vi "Main.vi"() -> ()   [LabVIEW 2017]
uses:
  Controls/Main_St.ctl
  Controls/Main_Loop_Data_Flow.ctl
  <vilib>/Utility/error.llb/DialogType.ctl
  <vilib>/Utility/config.llb/NI_LVConfig.lvlib
panel:
  in  "Recipe":bool
  in  "USER CREATER":bool
  in  "HARDWARE SETTING":bool
  in  "APPLICATION LAUNCH":bool
  in  "Login":bool
  out "Number of Monitor Connected":i32
  out "error out":errorcluster
  in  "Close":bool
  out "Machine Name":string
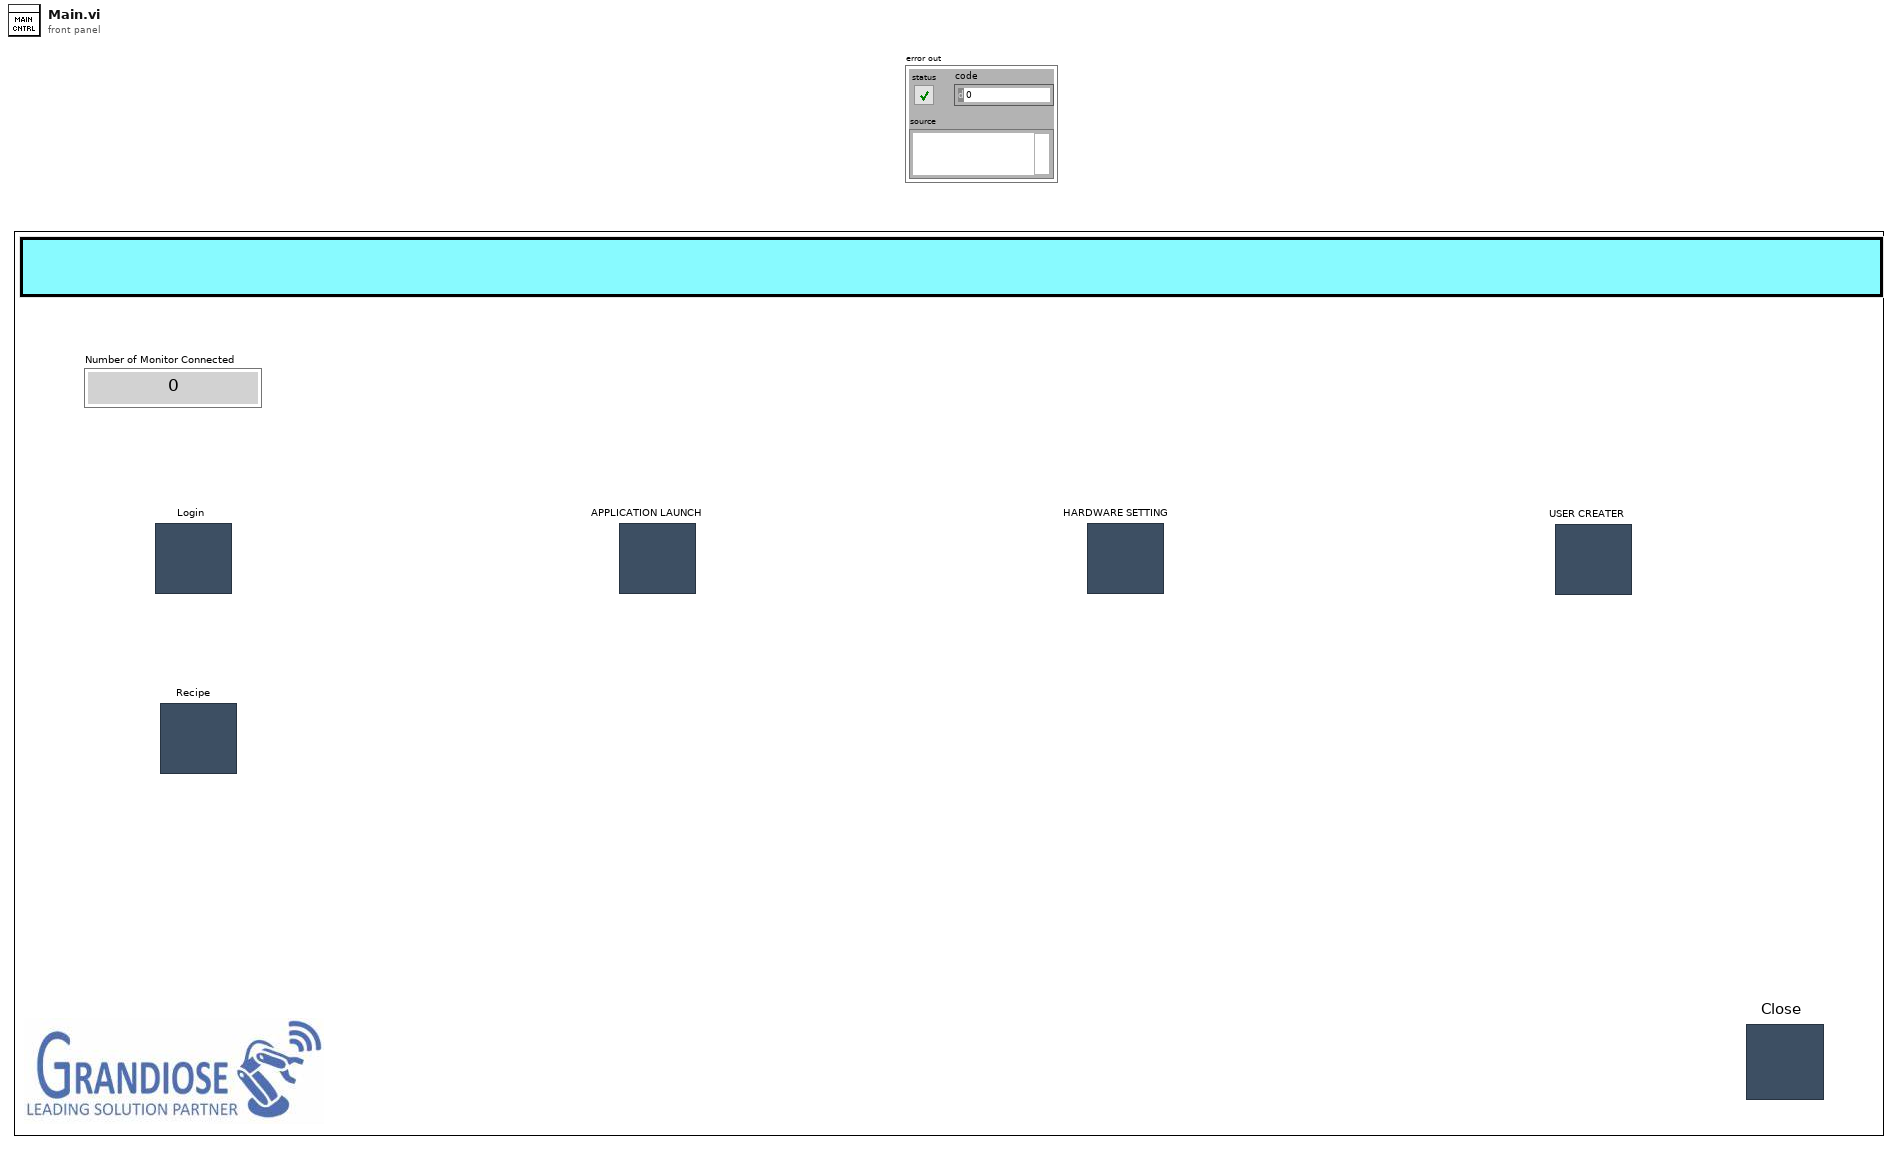
[diagram p1: front panel]
types:
  T1 = typedef "Main_Loop_Data_Flow.ctl" = cluster{"Hardware Setting":path, "Hardware":cluster{"Monitor Primary 1":u16, "Monitor 2":u16, "Monitor 3":u16, "Scanner IP":string, "Scanner 2":refnum<visa-resource-name>, "Scanner 3":refnum<visa-resource-name>, "Printer IP":string, "Printer 2":refnum<visa-resource-name>, "Printer 3":refnum<visa-resource-name>}, "SOP Path":path, "PNR Path":path, "PRN Data":string}
  T2 = typedef "Main_St.ctl" = enum16{"Int", "Int2", "Int3", "Wait", "Exit"}
  T3 = enum32{"Invalid", "Standard", "Closed", "Hidden", "Minimized", "Maximized"}
  T4 = typedef "DialogType.ctl" = u16
  T5 = enum8{"Enabled", "Disabled", "Disabled and Grayed Out"}
  T6 = enum32{"invalid app kind", "Development System", "Run Time System", "Student Edition", "Embedded LabVIEW", "Evaluation", "Custom"}
  T7 = cluster{"Monitor Primary 1":u16, "Monitor 2":u16, "Monitor 3":u16, "Scanner IP":string, "Scanner 2":refnum<visa-resource-name>, "Scanner 3":refnum<visa-resource-name>, "Printer IP":string, "Printer 2":refnum<visa-resource-name>, "Printer 3":refnum<visa-resource-name>}
  T8 = typedef "LVAllMonitorsDisplayTypeDef.ctl" = cluster{"Bounds":cluster{"Left":i16, "Top":i16, "Right":i16, "Bottom":i16}, "Depth":i16}[]
  T9 = typedef "NI_LVConfig.lvlib/Config Data RefNum.ctl" = refnum<k1>
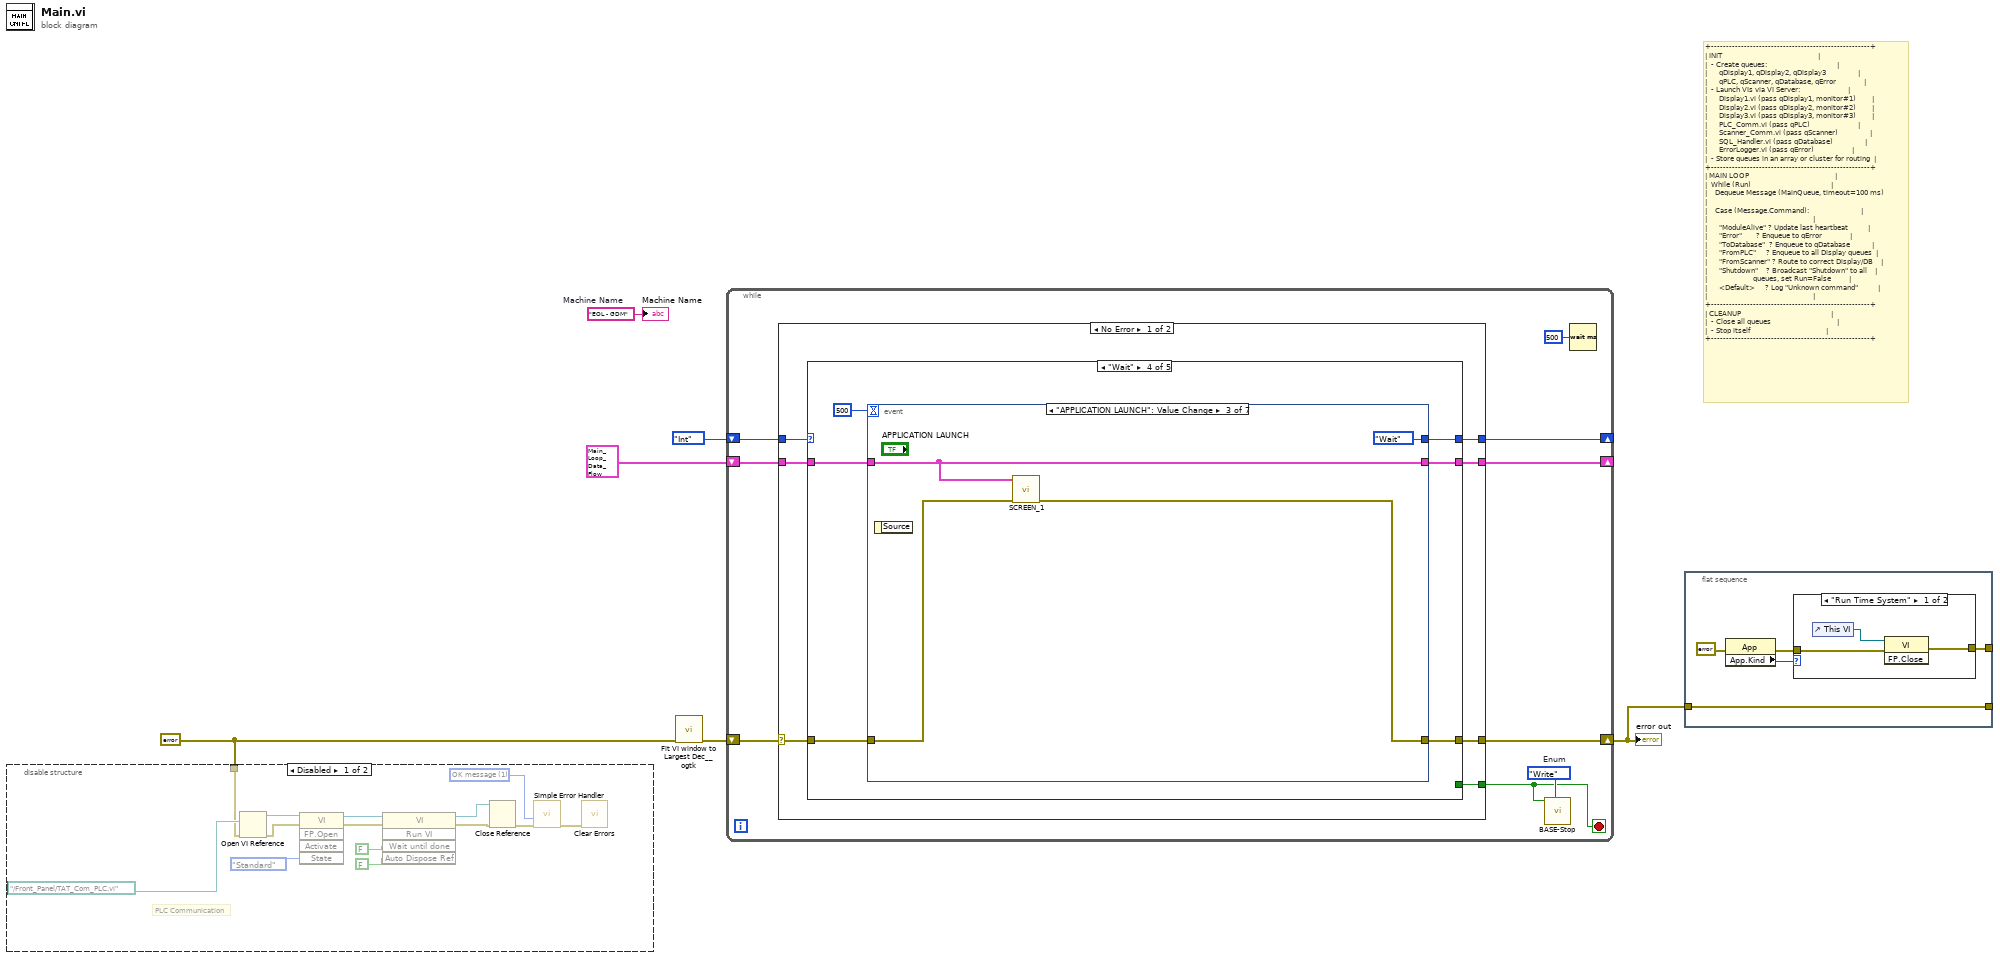
[diagram p0: block diagram]
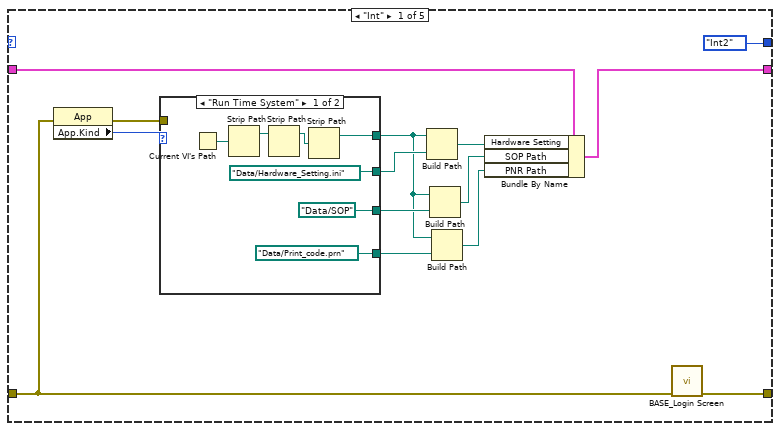
[diagram p4: hidden frame]
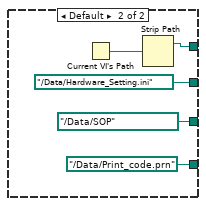
[diagram p5: hidden frame]
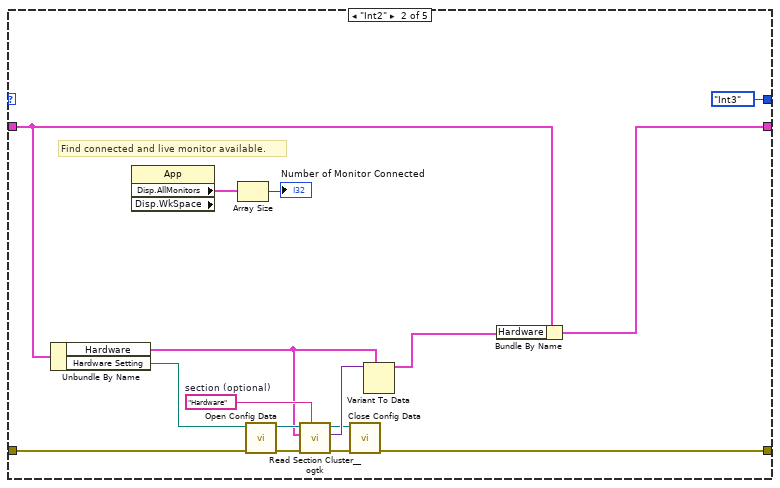
[diagram p6: hidden frame]
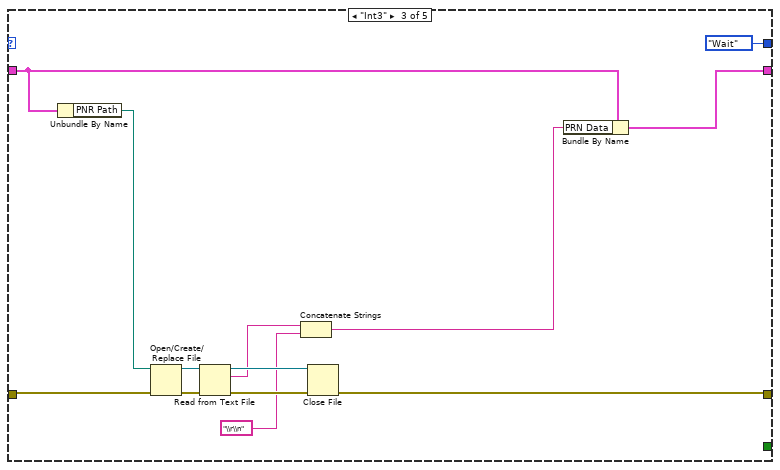
[diagram p7: hidden frame]
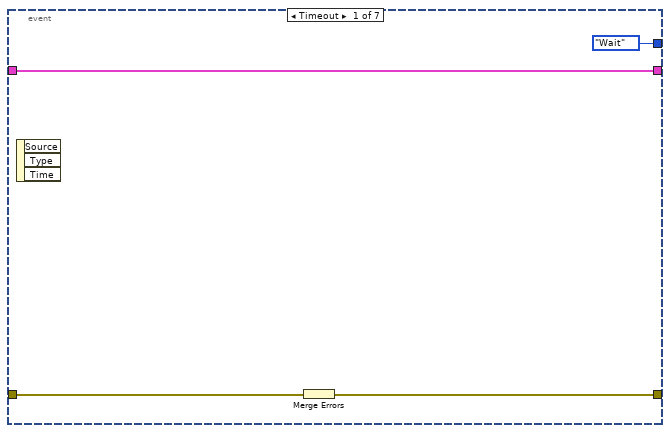
[diagram p8: hidden frame]
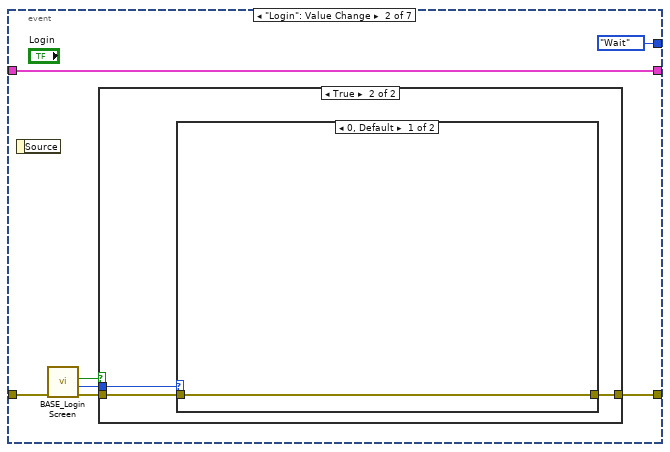
[diagram p9: hidden frame]
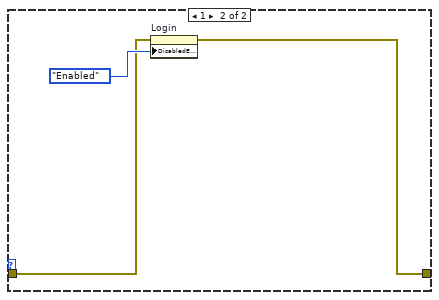
[diagram p11: hidden frame]
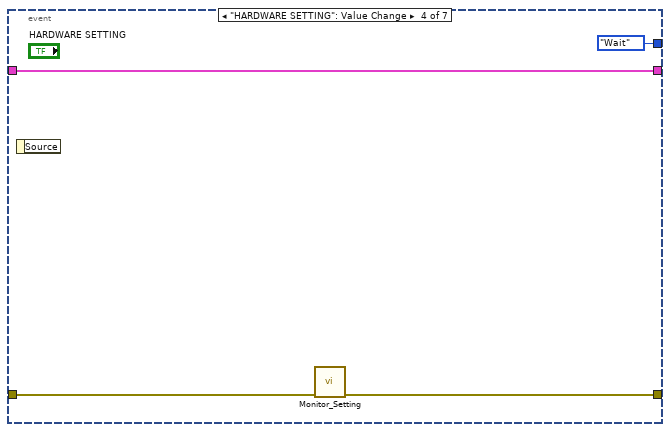
[diagram p12: hidden frame]
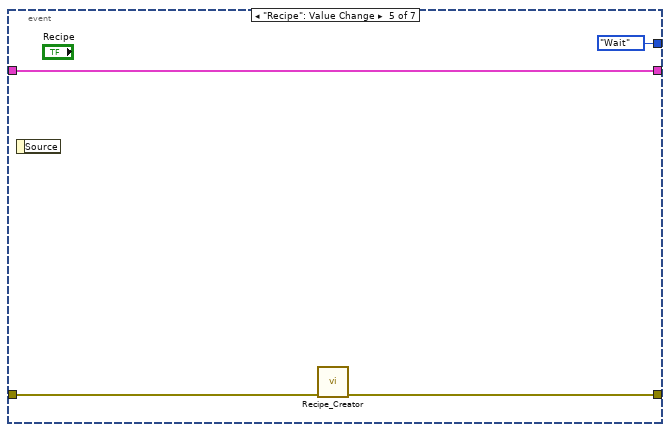
[diagram p13: hidden frame]
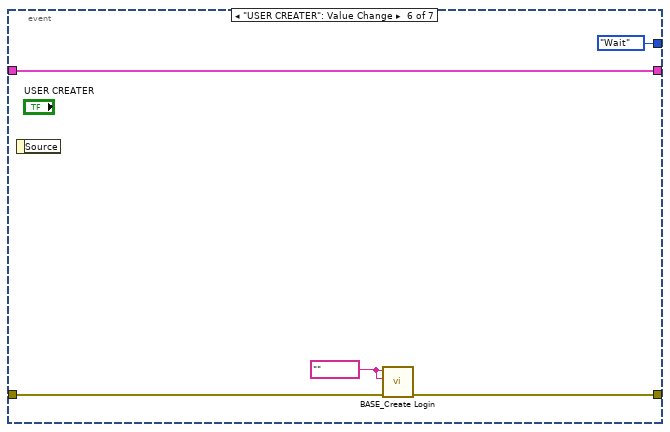
[diagram p14: hidden frame]
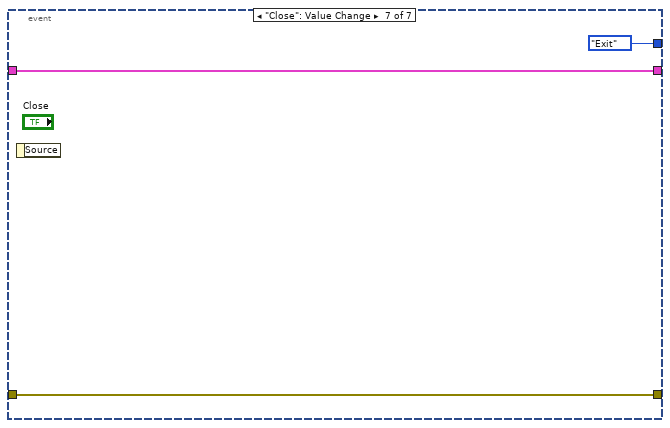
[diagram p15: hidden frame]
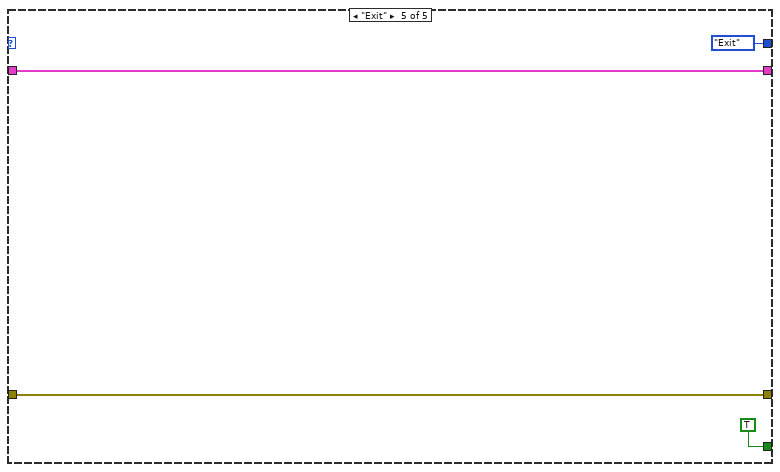
[diagram p16: hidden frame]
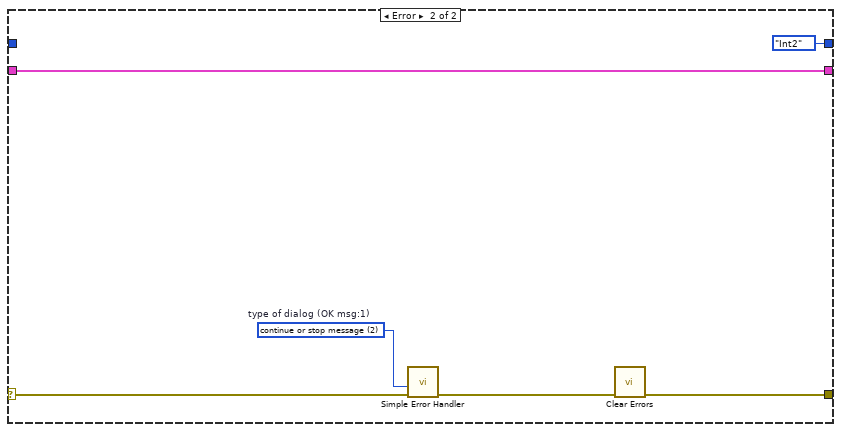
[diagram p17: hidden frame]
diagram:
  w3 = errorcluster {"status"=FALSE, "code"=0, "source"=""} ("error in (no error)")
  w6 = "EOL - GDM"  # Machine Name
  # "+-----------------------------------------------------+\n| INIT                                                |\n|  - Create queues:                                   |\n|      qDisplay1, qDisplay2, qDisplay3                |\n|      qPLC, qScanner, qDatabase, qError              |\n|  - Launch VIs via VI Server:                        |\n|      Display1.vi (pass qDisplay1, monitor#1)        |\n|      Display2.vi (pass qDisplay2, monitor#2)        |\n|      Display3.vi (pass qDisplay3, monitor#3)        |\n|      PLC_Comm.vi (pass qPLC)                        |\n|      Scanner_Comm.vi (pass qScanner)                |\n|      SQL_Handler.vi (pass qDatabase)                |\n|      ErrorLogger.vi (pass qError)                   |\n|  - Store queues in an array or cluster for routing  |\n+-----------------------------------------------------+\n| MAIN LOOP                                           |\n|  While (Run)                                        |\n|    Dequeue Message (MainQueue, timeout=100 ms)      |\n|    Case (Message.Command):                          |\n|                                                     |\n|      \"ModuleAlive\" ? Update last heartbeat          |\n|      \"Error\"       ? Enqueue to qError              |\n|      \"ToDatabase\"  ? Enqueue to qDatabase           |\n|      \"FromPLC\"     ? Enqueue to all Display queues  |\n|      \"FromScanner\" ? Route to correct Display/DB    |\n|      \"Shutdown\"    ? Broadcast \"Shutdown\" to all    |\n|                       queues, set Run=False         |\n|      <Default>     ? Log \"Unknown command\"          |\n|                                                     |\n+-----------------------------------------------------+\n| CLEANUP                                             |\n|  - Close all queues                                 |\n|  - Stop itself                                      |\n+-----------------------------------------------------+"
  n1 = disable-structure shown="Disabled" {
    disable-tunnel: w3 -> [w8 _]
    frame Disabled {
      w10 = T4 1 items=["no dialog", "OK message", "continue or stop message", "OK message + warnings", "continue/stop + warnings"] ("type of dialog (OK msg:1)")
      # "PLC Communication"
      n2 = Open VI Reference(vi path=path "../Front_Panel/TAT_Com_PLC.vi", error in (no error)=w8) -> (vi reference=w17:refnum<vi>, error out=w18:errorcluster)  [unwired: 4 in]
      n3 = invoke class="VI" method="FP.Open"(reference=w17, error in=w18, "State"=T3."Standard") -> (reference out=w20:refnum<vi>, error out=w19:errorcluster)  [unwired: 2 in, 3 out]
      n4 = invoke class="VI" method="Run VI"(reference=w20, error in=w19, "Wait until done"=FALSE ("Wait Until Done"), "Auto Dispose Ref"=FALSE ("Auto Dispose Reference")) -> (reference out=w7:refnum<vi>, error out=w16:errorcluster)  [unwired: 1 in, 3 out]
      n5 = Close Reference(reference=w7, error in (no error)=w16) -> (error out=w11:errorcluster)
      n6 = call <vilib>:"Simple Error Handler.vi"("type of dialog (OK msg:1)"=w10, "error in (no error)"=w11) -> ("error out"=w9:errorcluster)  [unwired: 3 in, 4 out]
      n7 = call <vilib>:"Clear Errors.vi"("error in (no error)"=w9) -> ()  [unwired: 5 in, 2 out]
    }
    frame Enabled {
    }
  }
  n8 = call <userlib>:"Fit VI window to Largest Dec__ogtk.vi"("error in (no error)"=w3) -> ("error out"=w5:errorcluster)  [unwired: 5 in, 1 out]
  n9 = while {
    shift-right: [w27] -> w1
    shift-left: w5 -> [w28]
    shift-right: [w23] -> _
    shift-left: Main_St."Int" -> [w26]
    shift-right: [w24] -> _
    shift-left: T1 {"Hardware Setting"=path "", "Hardware"={"Monitor Primary 1"=1, "Monitor 2"=2, "Monitor 3"=3, "Scanner IP"="", "Scanner 2"="", "Scanner 3"="", "Printer IP"="", "Printer 2"="", "Printer 3"=""}, "SOP Path"=path "", "PNR Path"=path "", "PRN Data"=""} -> [w25]
    stop <- w21 stop-if-true
    w22 = enum16{"Read", "Write"}."Write"  # Enum
    n10 = case shown="No Error" w28 {
      selector: w28 -> [w36 w146]
      tunnel: [w35 w141] -> w27
      tunnel: w26 -> [w34 _]
      tunnel: w25 -> [w33 w143]
      tunnel: [w32 w143] -> w24
      tunnel: [w31 Main_St."Int2"] -> w23
      tunnel: [w30 _] -> w21
      frame No Error {
        n11 = case shown="\"Wait\"" w34 {
          tunnel: w36 -> [w44 w71 w84 w97 w137]
          tunnel: [w43 w69 w83 w96 w137] -> w35
          tunnel: w33 -> [w47 w67 w81 w93 w139]
          tunnel: [w46 w66 w80 w92 w139] -> w32
          tunnel: [Main_St."Int2" Main_St."Int3" Main_St."Wait" w95 Main_St."Exit"] -> w31
          tunnel: [_ _ _ _ TRUE] -> w30
          frame "Int" {
            n12 = property class="App"(error in=w44) -> (error out=w50:errorcluster, "App.Kind"=w48:T6)  [unwired: 1 in, 1 out]
            n13 = case shown="\"Run Time System\"" w48 {
              tunnel: [path "Data/Hardware_Setting.ini" ("path") path "../Data/Hardware_Setting.ini" ("path")] -> w49
              tunnel: [w53 w60] -> w38
              tunnel: w50 -> [_ _]
              tunnel: [path "Data/SOP" ("path") path "../Data/SOP" ("path")] -> w41
              tunnel: [path "Data/Print_code.prn" ("path") path "../Data/Print_code.prn" ("path")] -> w39
              frame "Run Time System" {
                n14 = Current VI's Path() -> (path=w56:path)
                n15 = Strip Path(path=w56) -> (stripped path=w55:path)  [unwired: 1 out]
                n16 = Strip Path(path=w55) -> (stripped path=w54:path)  [unwired: 1 out]
                n17 = Strip Path(path=w54) -> (stripped path=w53:path)  [unwired: 1 out]
              }
              frame Default {
                n18 = Current VI's Path() -> (path=w61:path)
                n19 = Strip Path(path=w61) -> (stripped path=w60:path)  [unwired: 1 out]
              }
            }
            n20 = Build Path(base path=w38, name or relative path=w49) -> (appended path=w42:path)
            n21 = Build Path(base path=w38, name or relative path=w41) -> (appended path=w40:path)
            n22 = Build Path(base path=w38, name or relative path=w39) -> (appended path=w37:path)
            n23 = Bundle By Name(cluster=w47, "Hardware Setting"=w42, "SOP Path"=w40, "PNR Path"=w37) -> (w46:T1)
            n24 = call "BASE_Login Screen.vi"("Error In"=w44) -> ("error out"=w43:errorcluster)  [unwired: 7 in, 3 out]
          }
          frame "Int2" {
            w72 = "Hardware"  # section (optional)
            # "Find connected and live monitor available."
            n25 = Unbundle By Name(w67) -> ("Hardware"=w65:T7, "Hardware Setting"=w70:path)
            n26 = property class="App" props=["Disp.AllMonitors", "Disp.WkSpace"]() -> ("Disp.AllMonitors"=w64:T8)  [unwired: 2 in, 3 out]
            n27 = Array Size(array=w64) -> (size(s)=→"Number of Monitor Connected":i32)
            n28 = call <vilib>:"Open Config Data.vi"("error in (no error)"=w71, "configuration file path"=w70) -> ("error out"=w73:errorcluster, "refnum"=w76:T9)  [unwired: 7 in, 1 out]
            n29 = call <userlib>:"Read Section Cluster__ogtk.vi"("section (optional)"=w72, "error in (no error)"=w73, "Section Formatted Cluster Type"=w65, "refnum"=w76) -> ("error out"=w74:errorcluster, "Section Formatted Cluster"=w77:variant, "dup refnum"=w75:T9)  [unwired: 3 in, 2 out]
            n30 = call <vilib>:"Close Config Data.vi"("error in (no error)"=w74, "refnum"=w75) -> ("error out"=w69:errorcluster)  [unwired: 8 in, 1 out]
            n31 = Variant To Data(type=w65, Variant=w77) -> (data=w68:T7)  [unwired: 1 in, 1 out]
            n32 = Bundle By Name(cluster=w67, "Hardware"=w68) -> (w66:T1)
          }
          frame "Int3" {
            n33 = Unbundle By Name(w81) -> ("PNR Path"=w82:path)
            n34 = Open/Create/Replace File(file path (use dialog)=w82, error in=w84) -> (refnum out=w89:refnum<file>, error out=w88:errorcluster)  [unwired: 4 in, 1 out]
            n35 = Read from Text File(file (use dialog)=w89, error in=w88) -> (refnum out=w90:refnum<file>, text=w85:string, error out=w87:errorcluster)  [unwired: 2 in, 1 out]
            n36 = Concatenate Strings(w85, "\\r\\n") -> (w79:string)
            n37 = Close File(refnum=w90, error in=w87) -> (error out=w83:errorcluster)  [unwired: 1 out]
            n38 = Bundle By Name(cluster=w81, "PRN Data"=w79) -> (w80:T1)
          }
          frame "Wait" {
            n39 = event shown="[2] \"APPLICATION LAUNCH\": Value Change" {
              selector: _ -> [_ _ _ _ _ _ _]
              dyn-events: _ -> [_ _ _ _ _ _ _]
              timeout: 500 -> [_ _ _ _ _ _ _]
              tunnel: w97 -> [w101 w107 w119 w122 w125 w131 w136]
              tunnel: [w100 w104 w118 w121 w126 w130 w136] -> w96
              tunnel: [Main_St."Wait" Main_St."Wait" Main_St."Wait" Main_St."Wait" Main_St."Wait" Main_St."Wait" Main_St."Exit"] -> w95
              tunnel: w93 -> [w98 w108 w117 w124 w128 w133 w134]
              tunnel: [w98 w108 w117 w124 w128 w133 w134] -> w92
              event Timeout {
                n40 = event-data() -> ()  [unwired: 1 in, 3 out]
                n41 = Merge Errors(w101) -> (w100:errorcluster)
              }
              event "Login": Value Change {
                n42 = event-data() -> ()  [unwired: 1 in, 1 out]
                n43 = call "BASE_Login Screen.vi"("Error In"=w107) -> ("error out"=w106:errorcluster, "Level"=w102:i32, "Login Done"=w103:bool)  [unwired: 7 in, 1 out]
                n44 = case shown="True" w103 {
                  tunnel: w106 -> [w109 w112]
                  tunnel: [w109 w111] -> w104
                  tunnel: w102 -> [_ w110]
                  frame False {
                  }
                  frame True {
                    n45 = case shown="0, Default" w110 {
                      tunnel: w112 -> [w113 w115]
                      tunnel: [w113 w114] -> w111
                      frame 0, Default {
                      }
                      frame 1 {
                        n46 = property on="Login" class="Bool"(error in=w115, "DisabledEnum"=T5."Enabled" ("Disabled")) -> (error out=w114:errorcluster)  [unwired: 1 in, 1 out]
                      }
                    }
                  }
                }
              }
              event "APPLICATION LAUNCH": Value Change {
                n47 = event-data() -> ()  [unwired: 1 in, 1 out]
                n48 = call "SCREEN_1.vi"("error in (no error)"=w119, "Main_Data_Flow"=w117) -> ("error OUT"=w118:errorcluster)  [unwired: 9 in]
              }
              event "HARDWARE SETTING": Value Change {
                n49 = event-data() -> ()  [unwired: 1 in, 1 out]
                n50 = call "Monitor_Setting.vi"("Error in"=w122) -> ("error out 2"=w121:errorcluster)  [unwired: 10 in]
              }
              event "Recipe": Value Change {
                n51 = event-data() -> ()  [unwired: 1 in, 1 out]
                n52 = call "Recipe_Creator.vi"("Error in"=w125) -> ("error out 2"=w126:errorcluster)  [unwired: 10 in]
              }
              event "USER CREATER": Value Change {
                w129 = ""
                n53 = event-data() -> ()  [unwired: 1 in, 1 out]
                n54 = call "BASE_Create Login.vi"("Error In"=w131, "Password"=w129, "User Name"=w129) -> ("error out"=w130:errorcluster)  [unwired: 6 in]
              }
              event "Close": Value Change {
                n55 = event-data() -> ()  [unwired: 1 in, 1 out]
              }
            }
          }
          frame "Exit" {
          }
        }
      }
      frame Error {
        w142 = T4 2 items=["no dialog", "OK message", "continue or stop message", "OK message + warnings", "continue/stop + warnings"]  # type of dialog (OK msg:1)
        n56 = call <vilib>:"Simple Error Handler.vi"("type of dialog (OK msg:1)"=w142, "error in (no error)"=w146) -> ("error out"=w145:errorcluster)  [unwired: 3 in, 4 out]
        n57 = call <vilib>:"Clear Errors.vi"("error in (no error)"=w145) -> ("error out"=w141:errorcluster)  [unwired: 5 in, 1 out]
      }
    }
    n58 = call "BASE-Stop.vi"("Enum"=w22, "Stop"=w21) -> ()  [unwired: 9 in, 1 out]
    n59 = Wait (ms)(milliseconds to wait=u32 500) -> ()  [unwired: 1 out]
  }
  "error out" <- w1
  n60 = flat-sequence {
    tunnel: [w148] -> _
    tunnel: [w147] -> _
    tunnel: w1 -> [w147]
    frame #0 {
      n61 = property class="App"(error in=errorcluster {"status"=FALSE, "code"=0, "source"=""} ("error in (no error)")) -> (error out=w150:errorcluster, "App.Kind"=w151:T6)  [unwired: 1 in, 1 out]
      n62 = case shown="\"Run Time System\"" w151 {
        tunnel: w150 -> [w153 w155]
        tunnel: [w152 w155] -> w148
        frame "Run Time System" {
          n63 = control-ref of="This VI"() -> (w154:refnum<vi>)
          n64 = invoke class="VI" method="FP.Close"(reference=w154, error in=w153) -> (error out=w152:errorcluster)  [unwired: 1 in, 2 out]
        }
        frame "Development System", Default {
        }
      }
    }
  }
  "Machine Name" <- w6
